vi "RichToFlatnixnet_grpc_DbGetDBCAttributeSizeRequest.vi"(5 "OutputClusterType":T1, 11 "InputCluster":T4) -> (3 "OutputCluster":T1)   [LabVIEW 2025, in "grpc-xnet_client.lvlib"]
uses:
  grpc-xnet_client.lvlib
  nixnet_grpc_DbGetDBCAttributeSizeRequest.ctl
  nixnet_grpc_DbGetDBCAttributeSizeRequest_mode_enum/nixnet_grpc_DbGetDBCAttributeSizeRequest_mode_enum.lvclass
  nidevice_grpc_Session.ctl
  nixnet_grpc_DbGetDBCAttributeSizeRequest_Flat.ctl
  nidevice_grpc_Session_Flat.ctl
  nixnet_grpc_GetDBCAttributeMode.ctl
  nixnet_grpc_DbGetDBCAttributeSizeRequest_mode_enum/nixnet_grpc_DbGetDBCAttributeSizeRequest_mode_enum.lvclass/nixnet_grpc_DbGetDBCAttributeSizeRequest_mode_enum.ctl
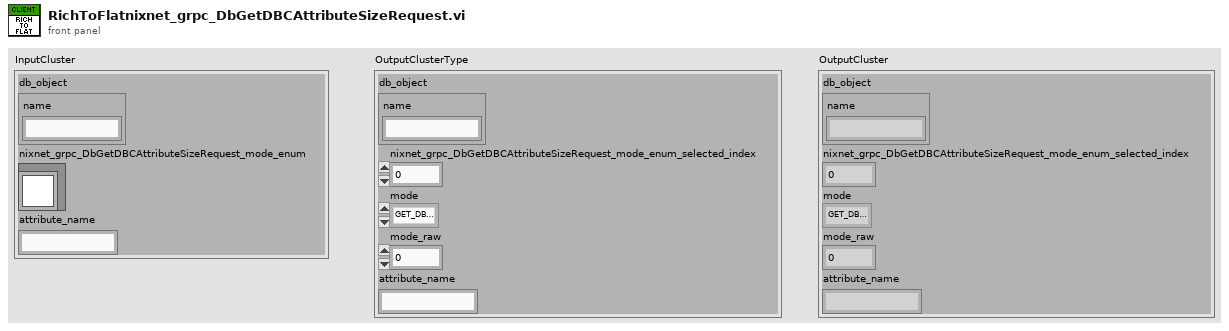
[diagram p1: front panel]
types:
  T1 = typedef "grpc-xnet_client.lvlib/nixnet_grpc_DbGetDBCAttributeSizeRequest_Flat.ctl" = cluster{"db_object":T2, "nixnet_grpc_DbGetDBCAttributeSizeRequest_mode_enum_selected_index":i32, "mode":T3, "mode_raw":u32, "attribute_name":string}
  T2 = typedef "grpc-xnet_client.lvlib/nidevice_grpc_Session_Flat.ctl" = cluster{"name":string}
  T3 = typedef "grpc-xnet_client.lvlib/nixnet_grpc_GetDBCAttributeMode.ctl" = enum32{"GET_DBC_ATTRIBUTE_MODE_ATTRIBUTE", "GET_DBC_ATTRIBUTE_MODE_ENUMERATION_LIST", "GET_DBC_ATTRIBUTE_MODE_ATTRIBUTE_LIST", "GET_DBC_ATTRIBUTE_MODE_VALUE_TABLE_LIST"}
  T4 = typedef "grpc-xnet_client.lvlib/nixnet_grpc_DbGetDBCAttributeSizeRequest.ctl" = cluster{"db_object":T5, "nixnet_grpc_DbGetDBCAttributeSizeRequest_mode_enum":refnum<class "nixnet_grpc_DbGetDBCAttributeSizeRequest_mode_enum.lvclass">, "attribute_name":string}
  T5 = typedef "grpc-xnet_client.lvlib/nidevice_grpc_Session.ctl" = cluster{"name":string}
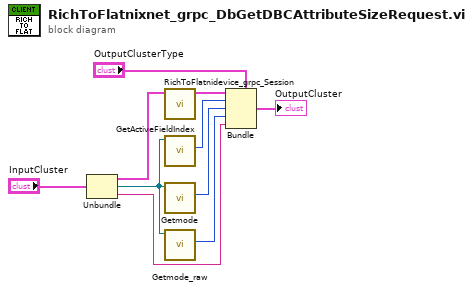
[diagram p0: block diagram]
diagram:
  n1 = Unbundle "Unbundle"("InputCluster") -> ("db_object"=w7:T5, "nixnet_grpc_DbGetDBCAttributeSizeRequest_mode_enum"=w5:refnum<class "nixnet_grpc_DbGetDBCAttributeSizeRequest_mode_enum.lvclass">, "attribute_name"=w1:string)
  n2 = call "RichToFlatnidevice_grpc_Session.vi"("InputCluster"=w7) -> ("OutputCluster"=w6:T2)  [unwired: 10 in]
  n3 = call "GetActiveFieldIndex.vi"("OneOfTemplate in"=w5) -> ("Active Field Index"=w4:i32)  [unwired: 8 in, 2 out]
  n4 = call "Getmode.vi"("OneOfTemplate in"=w5) -> ("Get_Val"=w3:T3)  [unwired: 8 in, 2 out]
  n5 = call "Getmode_raw.vi"("OneOfTemplate in"=w5) -> ("Get_Val"=w2:u32)  [unwired: 8 in, 2 out]
  n6 = Bundle "Bundle"(cluster="OutputClusterType", "db_object"=w6, "nixnet_grpc_DbGetDBCAttributeSizeRequest_mode_enum_selected_index"=w4, "mode"=w3, "mode_raw"=w2, "attribute_name"=w1) -> (→"OutputCluster":T1)
